vi "Trig Out Routing VI.vi"   [LabVIEW 2023]
uses:
  <vilib>/rvi/eio/common/nirviEmuTemplateMethod_errors.vi
  <vilib>/eio/EIONode/EIONode.xnode
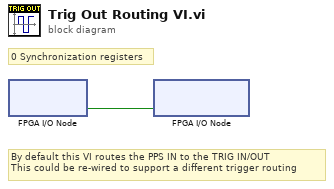
[diagram p0: block diagram]
diagram:
  # "By default this VI routes the PPS IN to the TRIG IN/OUT\nThis could be re-wired to support a different trigger routing"
  # "0 Synchronization registers"
  n1 = xnode "FPGA I/O Node"() -> ("PPS IN"=w1:bool)  [unwired: 1 in, 1 out]
  n2 = xnode "FPGA I/O Node"("TRIG OUT"=w1) -> ()  [unwired: 1 in, 1 out]
